vi "Handle Error.vi"(8 "error in (no error)":errorcluster, 11 "SoftwareSetup in":refnum<class "SoftwareSetup.lvclass">) -> (0 "error out":errorcluster, 2 "stop actor?":bool=TRUE, 3 "SoftwareSetup out":refnum<class "SoftwareSetup.lvclass">)   [LabVIEW 2019, in "SoftwareSetup.lvlib" / "SoftwareSetup.lvclass"]
uses:
  SoftwareSetup.lvclass
  SystemSetup/SystemSetup/SystemSetup.lvclass
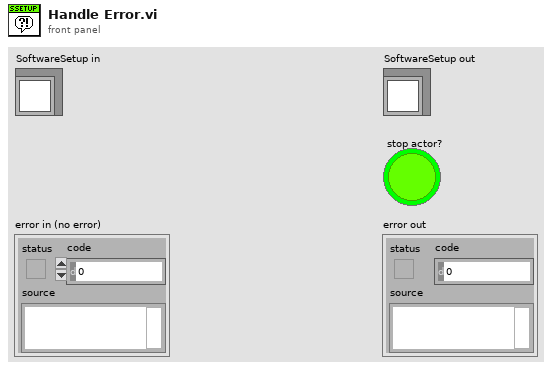
[diagram p1: front panel]
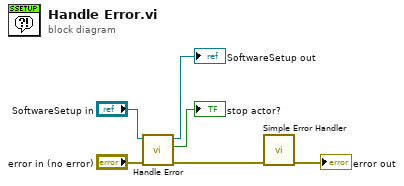
[diagram p0: block diagram]
diagram:
  n1 = call-parent "Handle Error.vi"("error in (no error)"="error in (no error)", "Actor in"="SoftwareSetup in") -> ("error out"=w6:errorcluster, "stop actor?"=→"stop actor?":bool, "Actor out"=→"SoftwareSetup out":refnum<class "SoftwareSetup.lvclass">)  [unwired: 7 in]
  n2 = call <vilib>:"Simple Error Handler.vi"("error in (no error)"=w6) -> ("error out"=→"error out":errorcluster)  [unwired: 4 in, 4 out]
